vi "Protection.vi"(11 "Diagnostic Data":T1) -> (3 "Diagnostic Data out":T1)   [LabVIEW 2014, in "MSX-E3711_dll.lvlib"]
doc: "Panel Frontal que se utiliza con la intención de configurar la protección de los transductores."
uses:
  MSX-E3711_dll.lvlib
  Typedef/Diagnostic Data.ctl
panel:
  in  "Cancelar":bool
  in  "Muestras Diag. Cycle":u32=10
  in  "Tolerancia Cycle":sgl=10.0 caption="Tolerancia % Cycle"
  in  "Tolerancia":sgl=10.0 caption="Tolerancia %"
  in  "OK":bool
  in  "Proteccion de Transductores":bool[][](array[boolean])
  # "1"
  # "2"
  # "3"
  # "4"
  # "5"
  # "6"
  # "7"
  # "8"
  # "9"
  # "10"
  # "11"
  # "12"
  # "13"
  # "14"
  # "15"
  # "16"
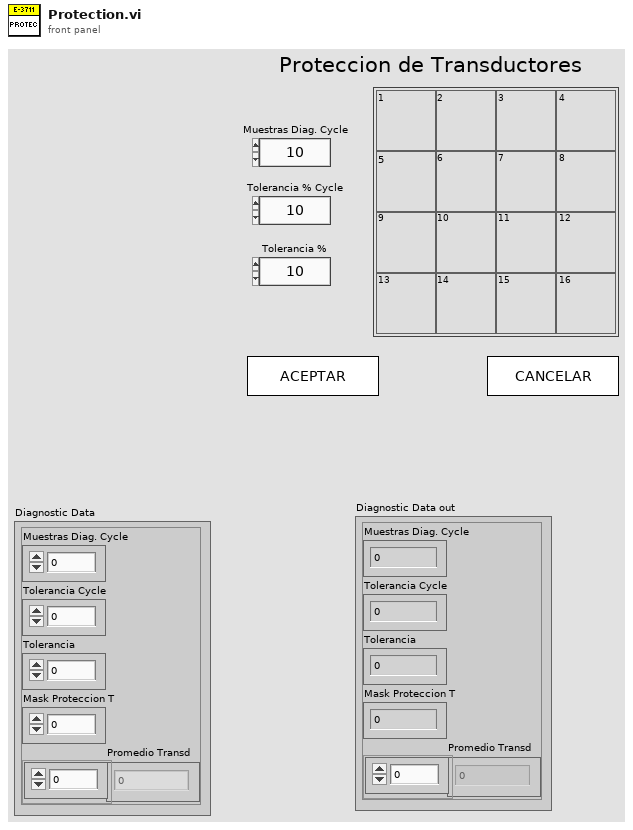
[diagram p1: front panel]
types:
  T1 = typedef "MSX-E3711_dll.lvlib/Diagnostic Data.ctl" = cluster{"Muestras Diag. Cycle":u32, "Tolerancia Cycle":sgl, "Tolerancia":sgl, "Mask Proteccion T":u64, "Promedio Transd":sgl[]}
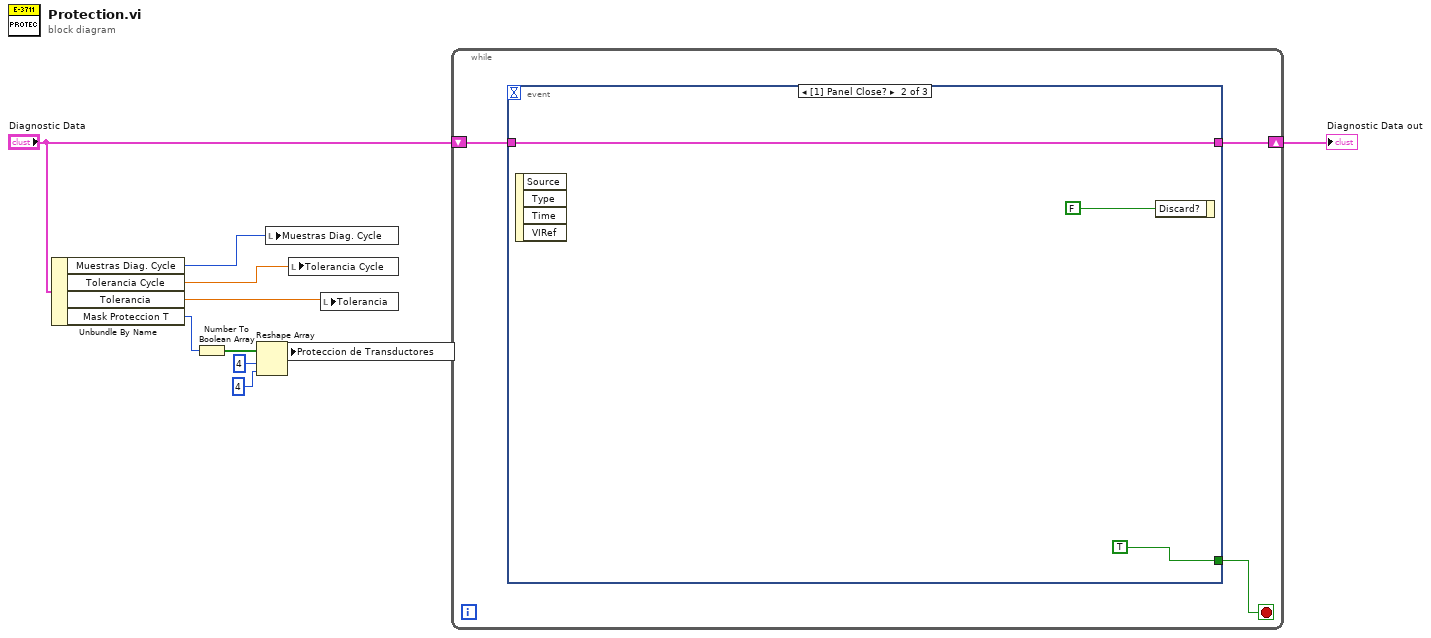
[diagram p0: block diagram]
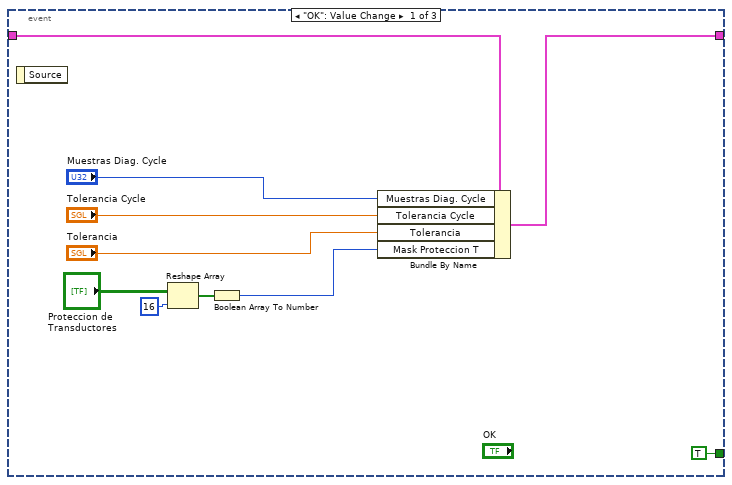
[diagram p2: hidden frame]
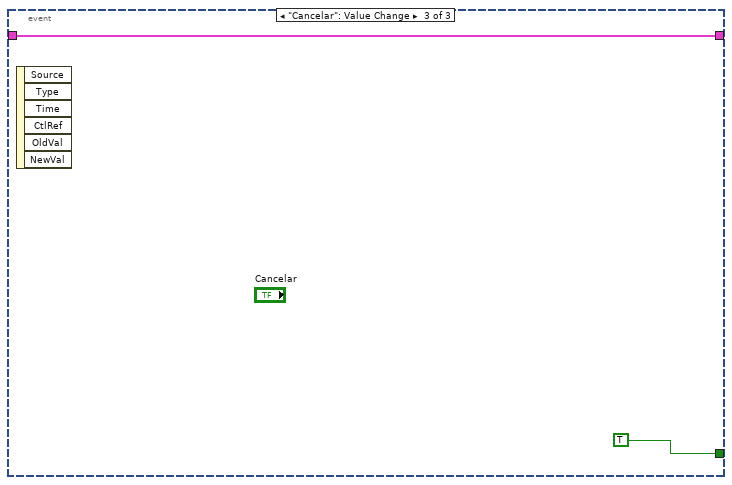
[diagram p3: hidden frame]
diagram:
  n1 = Unbundle By Name("Diagnostic Data") -> ("Muestras Diag. Cycle"=w8:u32, "Tolerancia Cycle"=w7:sgl, "Tolerancia"=w6:sgl, "Mask Proteccion T"=w5:u64)
  n2 = Number To Boolean Array(number=w5) -> (Boolean array=w4:bool[])
  n3 = Reshape Array(w4, 4 ("dimension size"), 4 ("dimension size")) -> (w3:bool[][])
  n4 = local write "Muestras Diag. Cycle"(w8) -> ()
  n5 = local write "Proteccion de Transductores"(w3) -> ()
  n6 = local write "Tolerancia Cycle"(w7) -> ()
  n7 = local write "Tolerancia"(w6) -> ()
  n8 = while {
    shift-right: [w11] -> w10
    shift-left: "Diagnostic Data" -> [w12]
    stop <- w13 stop-if-true
    n9 = event shown="[1] Panel Close?" {
      selector: _ -> [_ _ _]
      dyn-events: _ -> [_ _ _]
      timeout: _ -> [_ _ _]
      tunnel: [TRUE ("Discard?") TRUE ("Discard?") TRUE ("Discard?")] -> w13
      tunnel: w12 -> [w23 w24 w27]
      tunnel: [w22 w24 w27] -> w11
      event "OK": Value Change {
        n10 = event-data() -> ()  [unwired: 1 in, 1 out]
        n11 = Reshape Array("Proteccion de Transductores", 16 ("dimension size")) -> (w21:bool[])
        n12 = Boolean Array To Number(Boolean array=w21) -> (number=w15:u32)
        n13 = Bundle By Name(cluster=w23, "Muestras Diag. Cycle"="Muestras Diag. Cycle", "Tolerancia Cycle"="Tolerancia Cycle", "Tolerancia"="Tolerancia", "Mask Proteccion T"=w15) -> (w22:T1)
      }
      event Panel Close? {
        n14 = event-data() -> ()  [unwired: 1 in, 4 out]
        n15 = event-data("Discard?"=FALSE) -> ()  [unwired: 1 in, 1 out]
      }
      event "Cancelar": Value Change {
        n16 = event-data() -> ()  [unwired: 1 in, 6 out]
      }
    }
  }
  "Diagnostic Data out" <- w10
